vi "Coincidence Windows.vi"() -> ()   [LabVIEW 2016]
panel:
  in  "CRT-wide":i32=10
  in  "Planar":i32=5
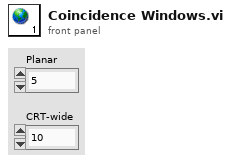
[diagram p1: front panel]
diagram:
